vi "Save_to_Project.vi"(8 "error in (no error)":errorcluster, 9 "index in":string, 10 "buildObject":T1, 11 "Class in":refnum<class "IB_Source_File.lvclass">) -> (0 "error out":errorcluster, 1 "index out":string, 2 "buildObject out":T1, 3 "Class out":refnum<class "IB_Source_File.lvclass">, 5 "saved?":bool)   [LabVIEW 2020, in "IB_Source_File.lvclass"]
uses:
  <vilib>/AppBuilder/IB_Classes/Source/File/IB_Source_File.lvclass
  <vilib>/AppBuilder/IB_Classes/Source/File/IB_Source_File.lvclass/IB_Source_File.ctl
  <vilib>/AppBuilder/IB_RW_Project/IB_RW_Project_PropBag_Action.ctl
  <vilib>/AppBuilder/IB_Classes/Shortcut/IB_Shortcut.lvclass
  <vilib>/AppBuilder/IB_Classes/Source/IB_Source.lvclass
  <resource>/Framework/Providers/API/ItemRef.ctl
  <vilib>/AppBuilder/IB_RW_Project/IB_RW_Project_Source_File_Data.ctl
panel:
  in  "data":T2
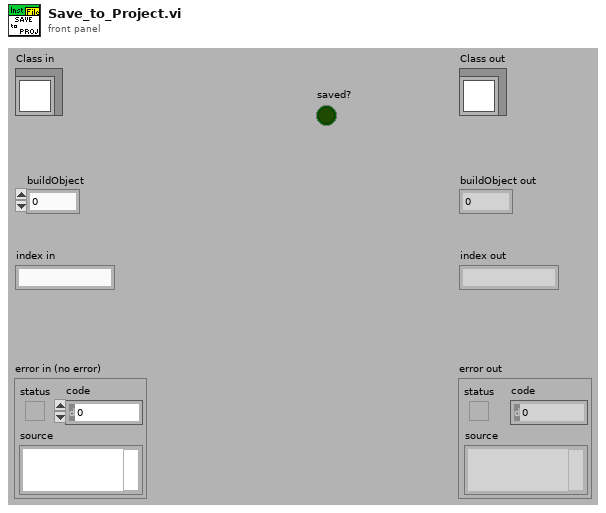
[diagram p1: front panel]
types:
  T1 = typedef "ItemRef.ctl" = u64
  T2 = typedef "IB_RW_Project_Source_File_Data.ctl" = cluster{"attributes":i16, "RegCOM":bool, "unlock":bool, "runEXE":bool, "cmdArg":string, "EXE_uninstall":bool, "CmdArg_uninstsall":string}
  T3 = typedef "IB_RW_Project_PropBag_Action.ctl" = enum16{"read", "write", "clear", "readPrevious", "writePrevious", "clearPrevious"}
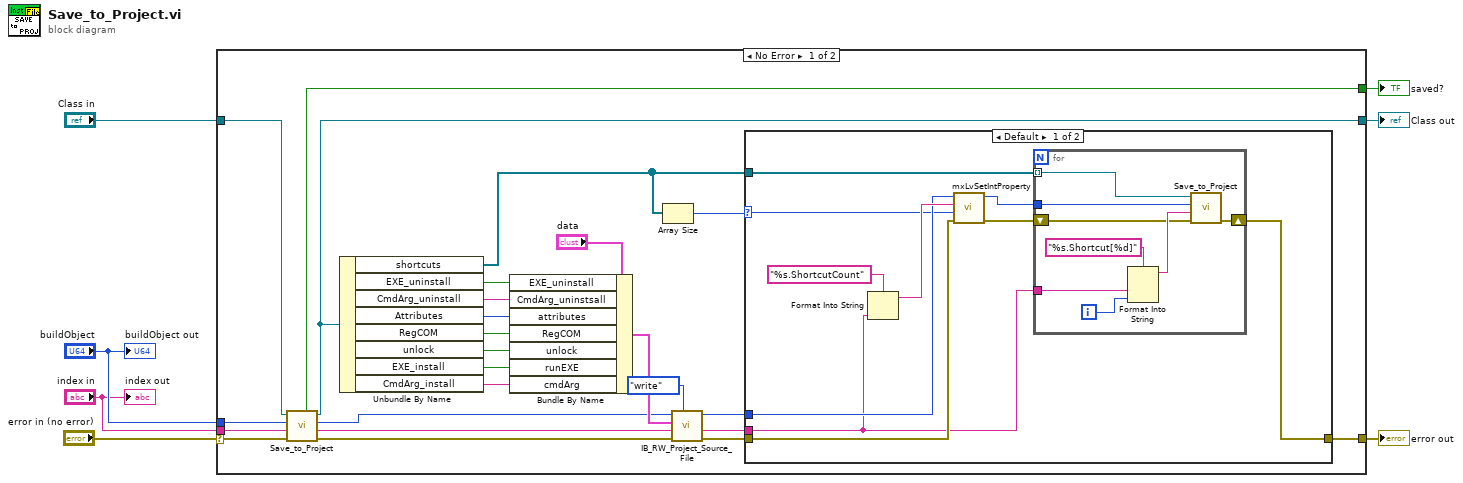
[diagram p0: block diagram]
diagram:
  n1 = case shown="No Error" "error in (no error)" {
    selector: "error in (no error)" -> [w29 w53]
    tunnel: [w15 w53] -> w7
    tunnel: [w26 w52] -> w6
    tunnel: "index in" -> [w32 _]
    tunnel: "buildObject" -> [w31 _]
    tunnel: "Class in" -> [w30 w52]
    tunnel: [w12 _] -> w1
    frame No Error {
      n2 = call-parent <vilib>:"Save_to_Project.vi"("error in (no error)"=w29, "index in"=w32, "buildObject"=w31, "Class in"=w30) -> ("error out"=w23:errorcluster, "index out"=w21:string, "buildObject out"=w19:T1, "Class out"=w26:refnum<class "IB_Source_File.lvclass">, "saved?"=w12:bool)  [unwired: 3 out]
      n3 = Unbundle By Name(w26) -> ("shortcuts"=w17:refnum<class "IB_Shortcut.lvclass">[], "EXE_uninstall"=w9:bool, "CmdArg_uninstall"=w8:string, "Attributes"=w24:i16, "RegCOM"=w27:bool, "unlock"=w28:bool, "EXE_install"=w11:bool, "CmdArg_install"=w10:string)
      n4 = Bundle By Name(cluster="data", "EXE_uninstall"=w9, "CmdArg_uninstsall"=w8, "attributes"=w24, "RegCOM"=w27, "unlock"=w28, "runEXE"=w11, "cmdArg"=w10) -> (w20:T2)
      n5 = Array Size(array=w17) -> (size(s)=w13:i32)
      n6 = call <vilib>:"IB_RW_Project_Source_File.vi"("action"=IB_RW_Project_PropBag_Action."write", "error in (no error)"=w23, "index in"=w21, "file in"=w20, "buildObject"=w19) -> ("error out"=w16:errorcluster, "index out"=w14:string, "buildObject out"=w18:T1)  [unwired: 4 out]
      n7 = case shown="Default" w13 {
        selector: w13 -> [w33 _]
        tunnel: w18 -> [w40 _]
        tunnel: w17 -> [w38 _]
        tunnel: w16 -> [w36 w51]
        tunnel: [w35 w51] -> w15
        tunnel: w14 -> [w34 _]
        frame Default {
          n8 = Format Into String(format string="%s.ShortcutCount", w34) -> (resulting string=w41:string)  [unwired: 2 in, 1 out]
          n9 = call <resource>:"mxLvSetIntProperty.vi"("error in"=w36, "Value (0)"=w33, "Tag"=w41, "Item"=w40) -> ("error out"=w37:errorcluster, "Item"=w39:T1)  [unwired: 1 in, 5 out]
          n10 = for {
            tunnel: w38 -> [w47] mode=indexing
            tunnel: w39 -> [w46]
            tunnel: w34 -> [w48]
            shift-right: [w44] -> w35
            shift-left: w37 -> [w43]
            i -> [w49]
            n11 = Format Into String(format string="%s.Shortcut[%d]", w48, w49) -> (resulting string=w45:string)  [unwired: 2 in, 1 out]
            n12 = call <vilib>:"Save_to_Project.vi"("error in (no error)"=w43, "index in"=w45, "buildObject"=w46, "IB_Shortcut in"=w47) -> ("error out"=w44:errorcluster)  [unwired: 7 out]
          }
        }
        frame 0 {
        }
      }
    }
    frame Error {
    }
  }
  "error out" <- w7
  "Class out" <- w6
  "saved?" <- w1
  "buildObject out" <- "buildObject"
  "index out" <- "index in"
